vi "saving graphs.vi"() -> ()   [LabVIEW 2018]
uses:
  <vilib>/Utility/file.llb/Write Delimited Spreadsheet (DBL).vi
  <vilib>/Utility/file.llb/Read Delimited Spreadsheet (DBL).vi
panel:
  out "Waveform Graph 2":dbl[][](graph)
  in  "file path (dialog if empty) 2":path
  in  "file path (dialog if empty)":path
  out "Waveform Graph":dynamicdata(graph)
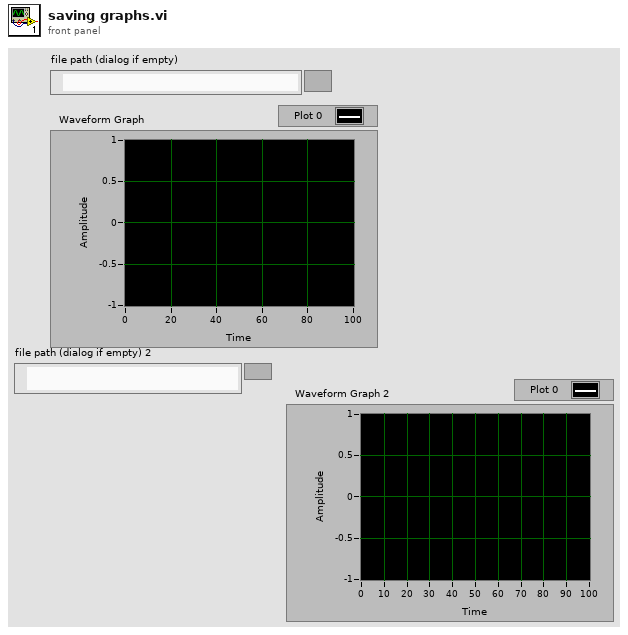
[diagram p1: front panel]
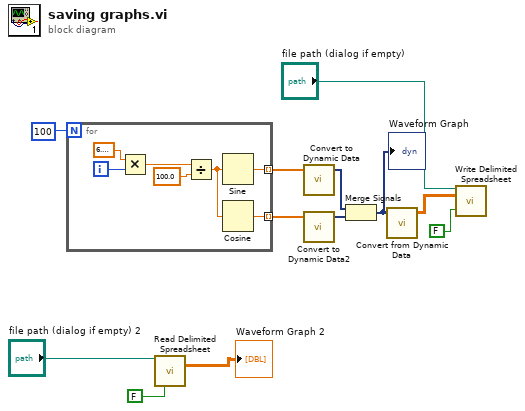
[diagram p0: block diagram]
diagram:
  n1 = for {
    N: 100 -> [_]
    tunnel: [w14] -> w11 mode=indexing
    tunnel: [w13] -> w9 mode=indexing
    i -> [w19]
    n2 = Multiply(x=6.283185307179586, y=w19) -> (x*y=w17:dbl)
    n3 = Divide(x=w17, y=100.0) -> (x/y=w15:dbl)
    n4 = Sine(x=w15) -> (sin(x)=w14:dbl)
    n5 = Cosine(x=w15) -> (cos(x)=w13:dbl)
  }
  n6 = call-poly <vilib>:"Read Delimited Spreadsheet.vi"("file path (dialog if empty)"="file path (dialog if empty) 2", "transpose? (F)"=FALSE) -> ("all rows"=→"Waveform Graph 2":dbl[][])  [unwired: 8 in, 5 out]
  n7 = call "Convert to Dynamic Data"("Array"=w11) -> ("Dynamic Data Type"=w10:dynamicdata)  [unwired: 3 in]
  n8 = call "Convert to Dynamic Data2"("Array"=w9) -> ("Dynamic Data Type"=w8:dynamicdata)  [unwired: 3 in]
  n9 = Merge Signals(w10, w8) -> (w6:dynamicdata)
  "Waveform Graph" <- w6
  n10 = call "Convert from Dynamic Data"("Dynamic Data Type"=w6) -> ("Array"=w5:dbl[][])  [unwired: 3 in]
  n11 = call-poly <vilib>:"Write Delimited Spreadsheet.vi"("file path (dialog if empty)"="file path (dialog if empty)", "2D data"=w5, "transpose? (no:F)"=FALSE) -> ()  [unwired: 11 in, 2 out]
